vi "TIFF-WriteHeader.vi"(8 "error in":errorcluster, 10 "[IN] byte order":T1(ring), 11 "[IN] refnum":refnum<file>) -> (0 "error out":errorcluster, 3 "[OUT] refnum":refnum<file>)   [LabVIEW 2020]
doc: "This VI writes a 8-byte tif header"
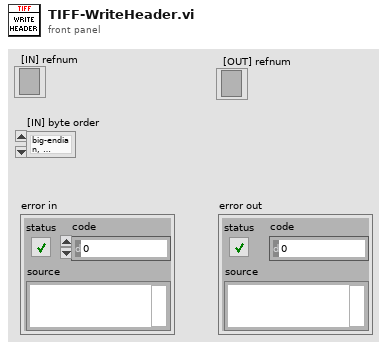
[diagram p1: front panel]
types:
  T1 = enum16{"big-endian, network order", "native, host order", "little-endian"}
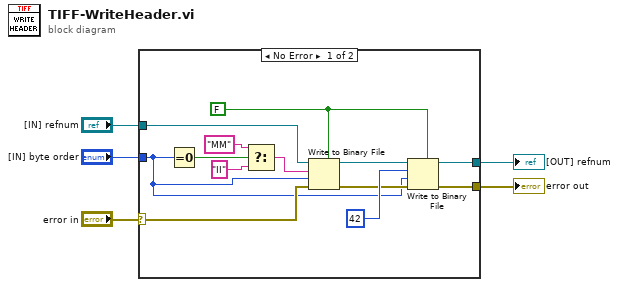
[diagram p0: block diagram]
diagram:
  n1 = case shown="No Error" "error in" {
    selector: "error in" -> [w9 w20]
    tunnel: [w13 w19] -> w5
    tunnel: [w10 w20] -> w4
    tunnel: "[IN] refnum" -> [w8 w19]
    tunnel: "[IN] byte order" -> [w6 _]
    frame No Error {
      w12 = FALSE ("prepend array or string size? (T)")
      n2 = Equal To 0?(x=w6) -> (x = 0?=w7:bool)
      n3 = Select(t="MM", s=w7, f="II") -> (s? t:f=w16:string)
      n4 = Write to Binary File(file (use dialog)=w8, data=w16, error in=w9, 5:w12, 9:w6) -> (refnum out=w15:refnum<file>, error out=w11:errorcluster)  [unwired: 1 in, 1 out]
      n5 = Write to Binary File(file (use dialog)=w15, data=u16 42, error in=w11, 5:w12, 9:w6) -> (refnum out=w13:refnum<file>, error out=w10:errorcluster)  [unwired: 1 in, 1 out]
    }
    frame Error {
    }
  }
  "[OUT] refnum" <- w5
  "error out" <- w4
